vi "Alarme_Pointing.vi"() -> ()   [LabVIEW 2018, in "client.lvlib"]
uses:
  client.lvlib
panel:
  out "IAG":bool
  in  "SAIR":bool
  out "160":bool
  # "APONTAMENTO"
  # "IAG"
  # "1,60"
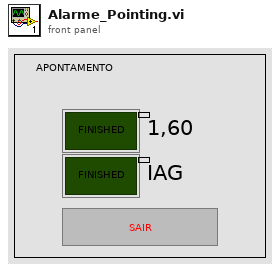
[diagram p1: front panel]
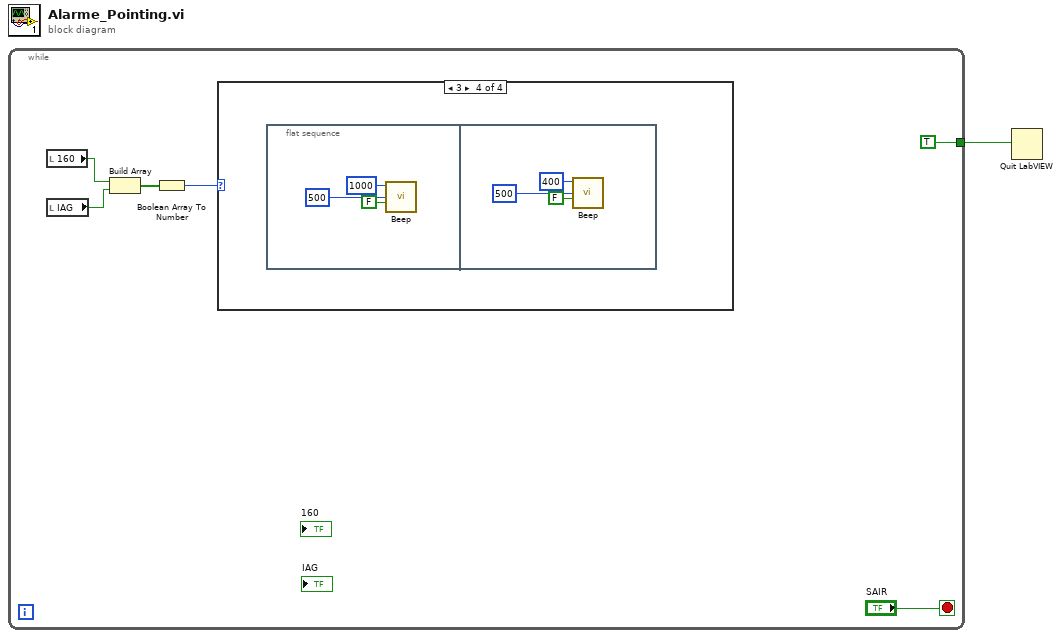
[diagram p0: block diagram]
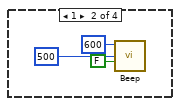
[diagram p3: hidden frame]
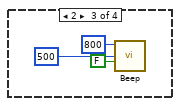
[diagram p4: hidden frame]
diagram:
  n1 = while {
    tunnel: [TRUE ("quit? (T)")] -> w1
    stop <- "SAIR" stop-if-true
    n2 = local read "160"() -> (w5:bool)
    n3 = local read "IAG"() -> (w4:bool)
    n4 = Build Array(w5, w4) -> (w3:bool[])
    n5 = Boolean Array To Number(Boolean array=w3) -> (number=w2:u32)
    n6 = case shown="3" w2 {
      frame 0, Default {
      }
      frame 1 {
        n7 = call <vilib>:"Beep.vi"("use system alert? (T)"=FALSE, "duration (msec)"=u32 500, "frequency (Hz)"=u32 600) -> ()  [unwired: 9 in]
      }
      frame 2 {
        n8 = call <vilib>:"Beep.vi"("use system alert? (T)"=FALSE, "duration (msec)"=u32 500, "frequency (Hz)"=u32 800) -> ()  [unwired: 9 in]
      }
      frame 3 {
        n9 = flat-sequence {
          frame #0 {
            n10 = call <vilib>:"Beep.vi"("use system alert? (T)"=FALSE, "duration (msec)"=u32 500, "frequency (Hz)"=u32 1000) -> ()  [unwired: 9 in]
          }
          frame #1 {
            n11 = call <vilib>:"Beep.vi"("use system alert? (T)"=FALSE, "duration (msec)"=u32 500, "frequency (Hz)"=u32 400) -> ()  [unwired: 9 in]
          }
        }
      }
    }
  }
  n12 = Quit LabVIEW(quit? (T)=w1) -> ()
